vi "Read Theme from Config.vi"(8 "error in":errorcluster) -> (0 "error out":errorcluster, 3 "Theme":bool)   [LabVIEW 2019, in "Panther Dashboard.lvlib"]
uses:
  Panther Dashboard.lvlib
  <vilib>/Utility/config.llb/NI_LVConfig.lvlib
  <vilib>/Utility/config.llb/Read Key (Boolean).vi
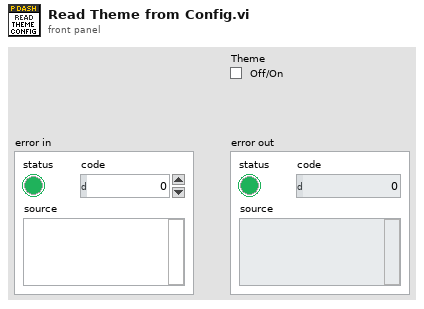
[diagram p1: front panel]
types:
  T1 = typedef "NI_LVConfig.lvlib/Config Data RefNum.ctl" = refnum<k1>
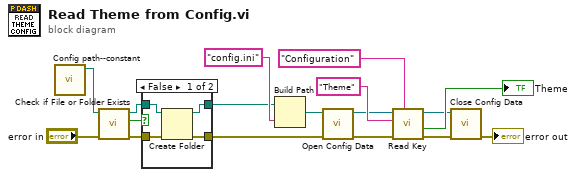
[diagram p0: block diagram]
diagram:
  n1 = call "Config path--constant.vi"() -> ("Config Path"=w5:path)  [unwired: 11 in]
  n2 = call <vilib>:"Check if File or Folder Exists.vi"("error in (no error)"="error in", "path"=w5) -> ("error out"=w16:errorcluster, "file or folder exists?"=w6:bool, "dup path"=w7:path)  [unwired: 7 in]
  n3 = case shown="False" w6 {
    tunnel: [w18 w22] -> w9
    tunnel: w7 -> [w19 w22]
    tunnel: w16 -> [w21 w23]
    tunnel: [w20 w23] -> w17
    frame False {
      n4 = Create Folder(path (use dialog)=w19, error in=w21) -> (created path=w18:path, error out=w20:errorcluster)  [unwired: 1 in, 1 out]
    }
    frame True {
    }
  }
  n5 = Build Path(base path=w9, name or relative path="config.ini") -> (appended path=w8:path)
  n6 = call <vilib>:"Open Config Data.vi"("error in (no error)"=w17, "configuration file path"=w8) -> ("error out"=w14:errorcluster, "refnum"=w2:T1)  [unwired: 7 in, 1 out]
  n7 = call-poly <vilib>:"Read Key.vi"("section"="Configuration", "error in (no error)"=w14, "key"="Theme", "refnum"=w2) -> ("error out"=w13:errorcluster, "value"=→"Theme":bool, "refnum out"=w1:T1)  [unwired: 4 in, 1 out]
  n8 = call <vilib>:"Close Config Data.vi"("error in (no error)"=w13, "refnum"=w1) -> ("error out"=→"error out":errorcluster)  [unwired: 8 in, 1 out]
